vi "IMAQdx Configure Acquisition.vi"(8 "error in":errorcluster, 9 "Number of Buffers":u32=1, 10 "Continuous?":T1, 11 "Session In":T2) -> (0 "error out":errorcluster, 3 "Session Out":T2)   [LabVIEW 2013, in "NI_Vision_Acquisition_Software.lvlib"]
doc: "Configures a low-level acquisition previously opened with IMAQdx Open Camera.vi. Specify the acquisition type with the Continuous? and Number of Buffers parameters. \n\nSnap Continuous = 0; Buffer Count = 1 \nSequence Continuous = 0; Buffer Count > 1 \nGrab Continuous = 1; Buffer Count > 1"
uses:
  NI_Vision_Acquisition_Software.lvlib
  IMAQdx.ctl
  IMAQdx Acquisition Mode.ctl
  niimaqdx.dll
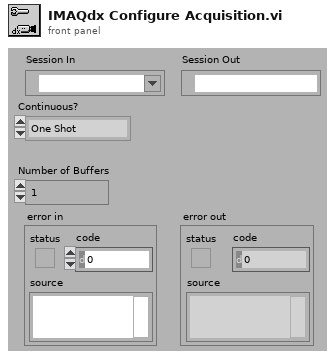
[diagram p1: front panel]
types:
  T1 = typedef "NI_Vision_Acquisition_Software.lvlib/IMAQdx Acquisition Mode.ctl" = enum32{"One Shot", "Continuous"}
  T2 = typedef "IMAQdx.ctl" = refnum<k21>
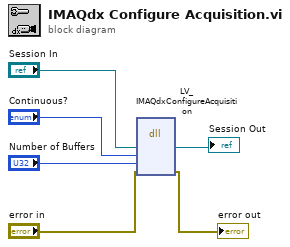
[diagram p0: block diagram]
diagram:
  n1 = dll-call lib="niimaqdx.dll" fn="LV_IMAQdxConfigureAcquisition"("Session In"="Session In", "continuous"="Continuous?", "bufferCount"="Number of Buffers", "error in"="error in") -> ("Session In"=→"Session Out":T2, "error in"=→"error out":errorcluster)  [unwired: 6 in, 2 out]
